vi "[Global]Script Number.vi"() -> ()   [LabVIEW 2015]
panel:
  in  "Script Number":i32=20
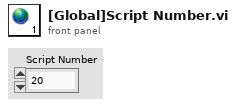
[diagram p1: front panel]
diagram:
